vi "closeLog.vi"(8 "error in (no error)":errorcluster, 11 "Model in":refnum<class "Model.lvclass">) -> (0 "error out":errorcluster, 3 "Model out":refnum<class "Model.lvclass">)   [LabVIEW 2015, in "Model.lvclass"]
uses:
  Model.lvclass
  Model.lvclass/Model.ctl
  <userlib>/Common/Log/Log/Log.lvclass
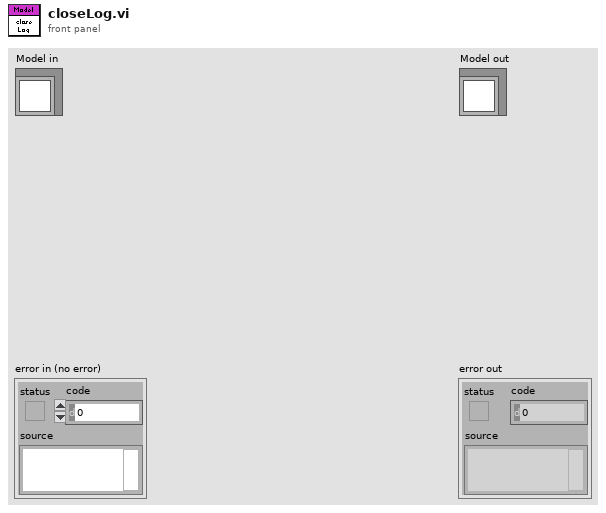
[diagram p1: front panel]
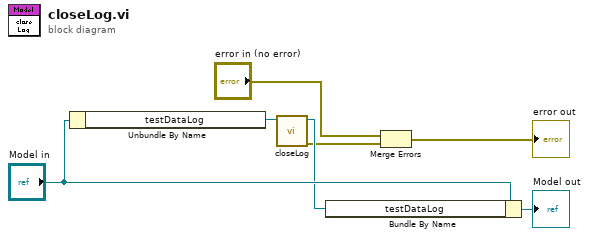
[diagram p0: block diagram]
diagram:
  n1 = Unbundle By Name("Model in") -> ("testDataLog"=w6:refnum<class "TestDataLog.lvclass">)
  n2 = call <userlib>:"closeLog.vi"("Logger in"=w6) -> ("error out"=w2:errorcluster, "Logger out"=w5:refnum<class "TestDataLog.lvclass">)  [unwired: 9 in]
  n3 = Bundle By Name(cluster="Model in", "testDataLog"=w5) -> (→"Model out":refnum<class "Model.lvclass">)
  n4 = Merge Errors("error in (no error)", w2) -> (→"error out":errorcluster)
